vi "set_query backlight.vi"(8 "error in (no error)":errorcluster, 9 "Query?":bool, 10 "Backlight (100 %)":u32=100 min=1 max=100 step=1, 11 "VISA resource name":refnum<visa-resource-name>) -> (0 "error out":errorcluster, 1 "Output backlight":string, 3 "VISA resource name out":refnum<visa-resource-name>)   [LabVIEW 2016]
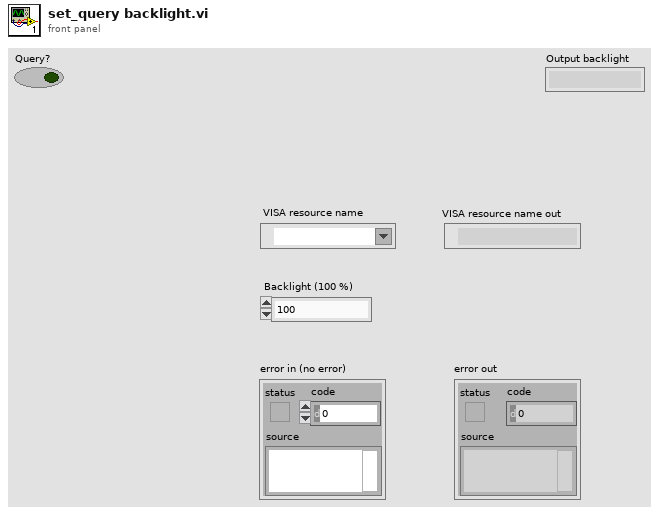
[diagram p1: front panel]
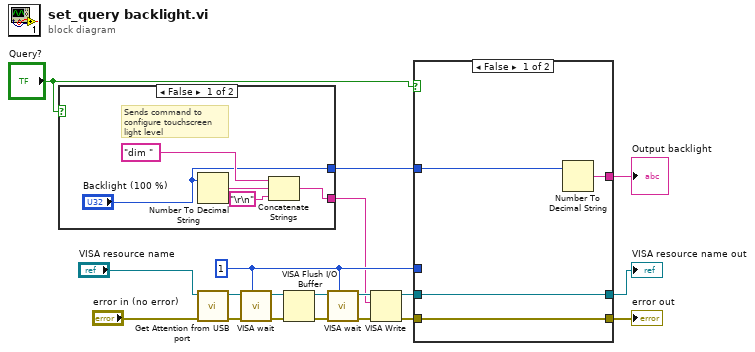
[diagram p0: block diagram]
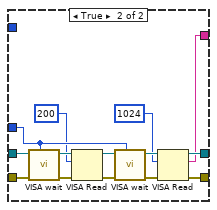
[diagram p2: hidden frame]
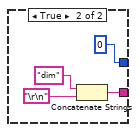
[diagram p3: hidden frame]
diagram:
  w5 = u32 1 ("milliseconds to wait")
  n1 = case shown="False" "Query?" {
    tunnel: [w21 w26] -> w4
    tunnel: ["Backlight (100 %)" u32 0 ("Force Level (100 %)")] -> w1
    frame False {
      # "Sends command to configure touchscreen light level"
      n2 = Number To Decimal String(number="Backlight (100 %)") -> (decimal integer string=w23:string)  [unwired: 1 in]
      n3 = Concatenate Strings("dim " ("command"), w23, "\r\n") -> (w21:string)
    }
    frame True {
      n4 = Concatenate Strings("dim" ("command"), "\r\n") -> (w26:string)
    }
  }
  n5 = call "Get Attention from USB port.vi"("error in (no error)"="error in (no error)", "VISA resource name"="VISA resource name") -> ("error out"=w16:errorcluster, "VISA resource name out"=w17:refnum<visa-resource-name>)  [unwired: 8 in]
  n6 = call <userlib>:"VISA wait.vi"("VISA resource name"=w17, "error in (no error)"=w16, "milliseconds to wait"=w5) -> ("VISA resource name out"=w14:refnum<visa-resource-name>, "error out"=w15:errorcluster)  [unwired: 6 in]
  n7 = VISA Flush I/O Buffer(VISA resource name=w14, error in (no error)=w15) -> (VISA resource name out=w9:refnum<visa-resource-name>, error out=w8:errorcluster)  [unwired: 1 in]
  n8 = call <userlib>:"VISA wait.vi"("VISA resource name"=w9, "error in (no error)"=w8, "milliseconds to wait"=w5) -> ("VISA resource name out"=w7:refnum<visa-resource-name>, "error out"=w6:errorcluster)  [unwired: 6 in]
  n9 = VISA Write(VISA resource name=w7, write buffer=w4, error in (no error)=w6) -> (VISA resource name out=w13:refnum<visa-resource-name>, error out=w12:errorcluster)  [unwired: 1 out]
  n10 = case shown="False" "Query?" {
    tunnel: w13 -> [w32 w46]
    tunnel: w12 -> [w31 w45]
    tunnel: [w32 w38] -> w11
    tunnel: [w31 w37] -> w10
    tunnel: w5 -> [_ w36]
    tunnel: [w29 w33] -> w2
    tunnel: w1 -> [w30 _]
    frame False {
      n11 = Number To Decimal String(number=w30) -> (decimal integer string=w29:string)  [unwired: 1 in]
    }
    frame True {
      n12 = call <userlib>:"VISA wait.vi"("VISA resource name"=w46, "error in (no error)"=w45, "milliseconds to wait"=w36) -> ("VISA resource name out"=w43:refnum<visa-resource-name>, "error out"=w44:errorcluster)  [unwired: 6 in]
      n13 = VISA Read(VISA resource name=w43, byte count=u32 200, error in (no error)=w44) -> (VISA resource name out=w42:refnum<visa-resource-name>, error out=w41:errorcluster)  [unwired: 2 out]
      n14 = call <userlib>:"VISA wait.vi"("VISA resource name"=w42, "error in (no error)"=w41, "milliseconds to wait"=w36) -> ("VISA resource name out"=w39:refnum<visa-resource-name>, "error out"=w40:errorcluster)  [unwired: 6 in]
      n15 = VISA Read(VISA resource name=w39, byte count=u32 1024, error in (no error)=w40) -> (VISA resource name out=w38:refnum<visa-resource-name>, read buffer=w33:string, error out=w37:errorcluster)  [unwired: 1 out]
    }
  }
  "VISA resource name out" <- w11
  "error out" <- w10
  "Output backlight" <- w2
